vi "Read Operation Mode.vi"(8 "error in (no error)":errorcluster, 11 "rqcBob in":refnum<class "rqcBob.lvclass">) -> (0 "error out":errorcluster, 2 "rqcBob Operation Mode":T1=enum."Channel Test", 3 "rqcBob out":refnum<class "rqcBob.lvclass">)   [LabVIEW 2019, in "rqcBob.lvclass"]
uses:
  rqcBob.lvclass
  Custom Controls/rqcBob Operation Mode.ctl
  rqcBob.lvclass/rqcBob.ctl
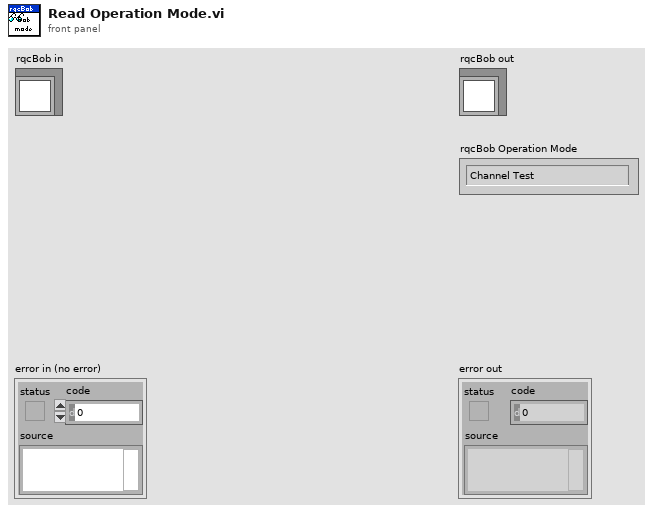
[diagram p1: front panel]
types:
  T1 = typedef "rqcBob.lvclass/rqcBob Operation Mode.ctl" = enum16{"Not Set", "Channel Test", "Key Distribution", "Modulation Level Test", "Window Test", "Delay Line Test", "Alice Modulation Level Test"}
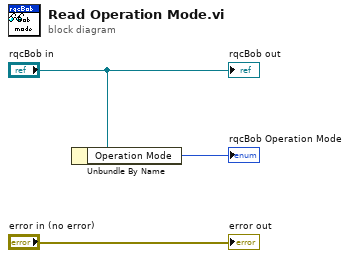
[diagram p0: block diagram]
diagram:
  n1 = Unbundle By Name("rqcBob in") -> ("Operation Mode"=→"rqcBob Operation Mode":T1)
  "error out" <- "error in (no error)"
  "rqcBob out" <- "rqcBob in"
